vi "fgt get sensor Calibration.vi"(8 "error in (no error)":errorcluster, 11 "sensorIndex":u32) -> (0 "error out":errorcluster, 3 "calibration out":T1=enum."H2O")   [LabVIEW 2020, in "fgt_SDK.lvlib"]
doc: "Get internal used calibration table by the sensor. Not supported by IPS."
uses:
  fgt_SDK.lvlib
  TypeDefs/fgt_SENSOR_CALIBRATION.ctl
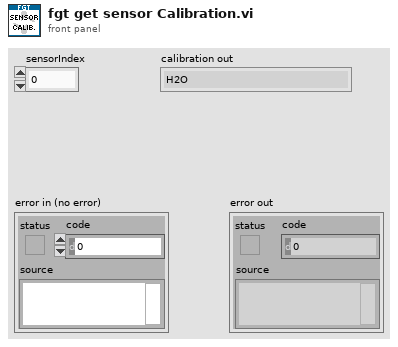
[diagram p1: front panel]
types:
  T1 = typedef "fgt_SDK.lvlib/fgt_SENSOR_CALIBRATION.ctl" = enum16{"None", "H2O", "IPA", "HFE", "FC40", "OIL"}
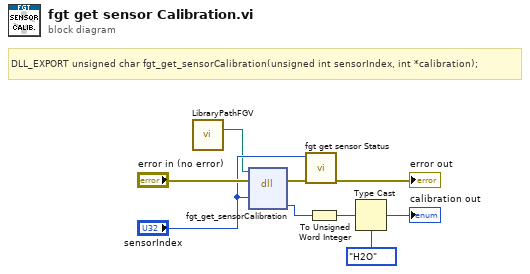
[diagram p0: block diagram]
diagram:
  # "DLL_EXPORT unsigned char fgt_get_sensorCalibration(unsigned int sensorIndex, int *calibration);"
  n1 = call "LibraryPathFGV.vi"() -> ("Path Out"=w1:path)  [unwired: 14 in, 1 out]
  n2 = dll-call lib="C:/Workspace/fgt-SDK/LabVIEW/dlls/fgt_SDK_*.*" fn="fgt_get_sensorCalibration"(path in=w1, error in="error in (no error)", "sensorIndex"="sensorIndex") -> (error out=w8:errorcluster, "calibration"=w5:i32)  [unwired: 4 in, 1 out]
  n3 = call "fgt get sensor Status.vi"("error in (no error)"=w8, "pressureIndex"="sensorIndex") -> ("error out"=→"error out":errorcluster)  [unwired: 9 in]
  n4 = To Unsigned Word Integer(number=w5) -> (unsigned 16bit integer=w4:u16)
  n5 = Type Cast(type=fgt_SENSOR_CALIBRATION."H2O" ("calibration out"), x=w4) -> (*(type *) &x=→"calibration out":T1)
